vi "Write Read Example.vi"() -> ()   [LabVIEW 2010]
uses:
  <vilib>/userDefined/High Color/nirio_resource_hc.ctl
  <vilib>/rvi/interface/nirviOpenFPGA/nirviOpenFPGA.xnode
  FPGA Bitfiles/Athena Brain.lvproj_FPGA Target 2_serial FPGA Main.vi.lvbitx
  serial FPGA Main.vi
  <vilib>/rvi/interface/nirviMethod/nirviMethod.xnode
  serial FPGA main reference type def.ctl
panel:
  out "VectorNav String":string
  in  "write?":bool
  in  "Data to write":string="\u0002\u0000\u0002\u0000 $4\b"
  out "error out":errorcluster
  out "LIDAR String":string
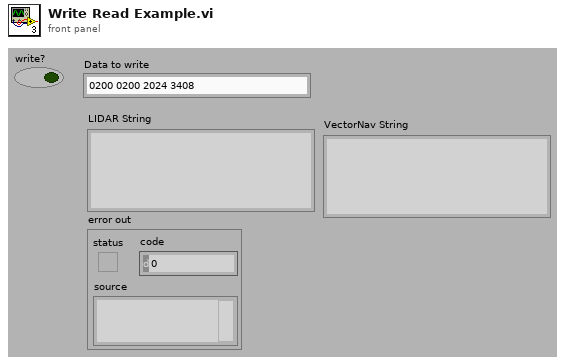
[diagram p1: front panel]
types:
  T1 = typedef "serial FPGA main reference type def.ctl" = refnum<k20>
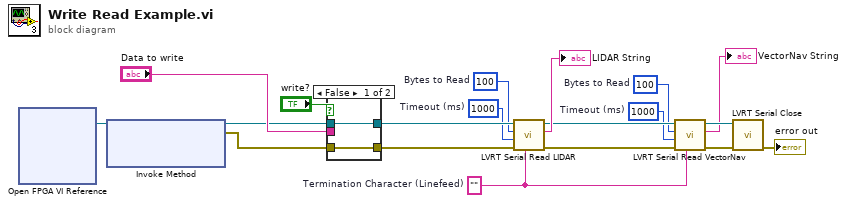
[diagram p0: block diagram]
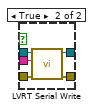
[diagram p2: hidden frame]
diagram:
  w3 = 1000  # Timeout (ms)
  w4 = u32 100  # Bytes to Read
  w2 = ""  # Termination Character (Linefeed)
  w13 = 1000  # Timeout (ms)
  w16 = u32 100  # Bytes to Read
  n1 = xnode "Open FPGA VI Reference"() -> ("FPGA VI Reference Out"=w11:T1)  [unwired: 2 in, 1 out]
  n2 = xnode "Invoke Method"("FPGA VI Reference In"=w11) -> ("FPGA VI Reference Out"=w10:T1, "error out"=w9:errorcluster)  [unwired: 1 in, 1 out]
  n3 = case shown="False" "write?" {
    tunnel: "Data to write" -> [_ w26]
    tunnel: [w20 w25] -> w18
    tunnel: [w21 w24] -> w17
    tunnel: w10 -> [w21 w23]
    tunnel: w9 -> [w20 w22]
    frame False {
    }
    frame True {
      n4 = call "LVRT Serial Write.vi"("error in (no error)"=w22, "String"=w26, "FPGA Main Ref"=w23) -> ("error out"=w25:errorcluster, "FPGA Main Ref Out"=w24:T1)  [unwired: 7 in]
    }
  }
  n5 = call "LVRT Serial Read LIDAR.vi"("Termination Character (Linefeed)"=w2, "error in (no error)"=w18, "Timeout (ms) (-1: no timeout)"=w13, "Bytes to Read"=w16, "FPGA Main Ref"=w17) -> ("error out"=w6:errorcluster, "LIDAR"=→"LIDAR String":string, "FPGA Main Ref Out"=w7:T1)  [unwired: 4 in]
  n6 = call "LVRT Serial Read VectorNav.vi"("Termination Character (Linefeed)"=w2, "error in (no error)"=w6, "Timeout (ms) (-1: no timeout)"=w3, "Bytes to Read"=w4, "FPGA Main Ref"=w7) -> ("error out"=w5:errorcluster, "VectorNav Data"=→"VectorNav String":string, "FPGA Main Ref Out"=w8:T1)  [unwired: 4 in]
  n7 = call "LVRT Serial Close.vi"("error out"=w5, "FPGA Main Ref"=w8) -> ("error out"=→"error out":errorcluster)  [unwired: 9 out]
